vi "Demo.vi"() -> ()   [LabVIEW 2020]
uses:
  Instantiate.vi
  Flex.lvlib
panel:
  out "Timed Out?":bool
  out "Count 2":i32
  out "Count 1":i32
  out "Slow i":i32
  out "Fast i":i32
  out "Lossy Fast Timeout":bool
  out "Timeout":bool
  in  "Publish Timeout":i32
  in  "Stop 4":bool
  in  "Stop 3":bool
  in  "Stop 2":bool
  in  "Stop 1":bool
  in  "Stop":bool
  out "Lossless Timeout":dbl(graph)
  out "Lossless":dbl(graph)
  out "Lossy Slow/Wait":dbl(graph)
  out "Lossy Fast":dbl(graph)
  in  "Publish Period mS":u32=10
  in  "Slide":dbl(slide)=5.0 scale=0.0..10.0
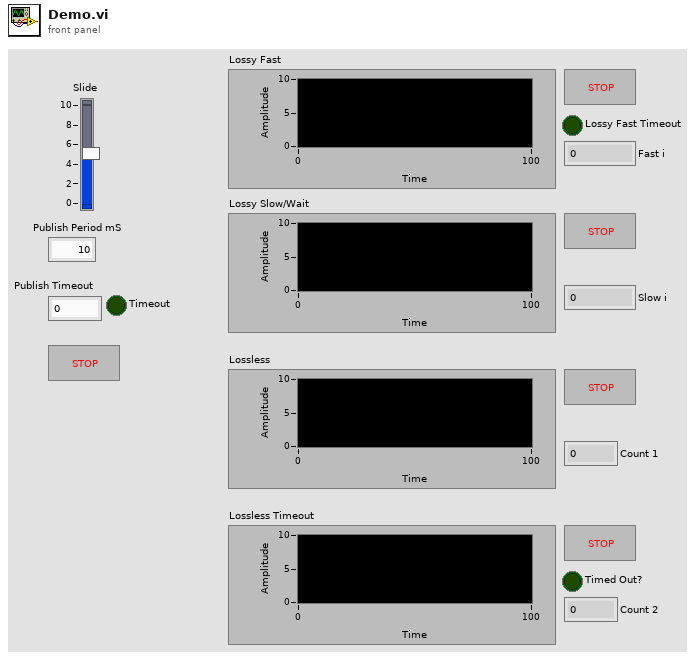
[diagram p1: front panel]
types:
  T1 = typedef "Flex.lvlib/))Channel.ctl" = refnum<queue>
  T2 = typedef "Flex.lvlib/Element.ctl" = dbl
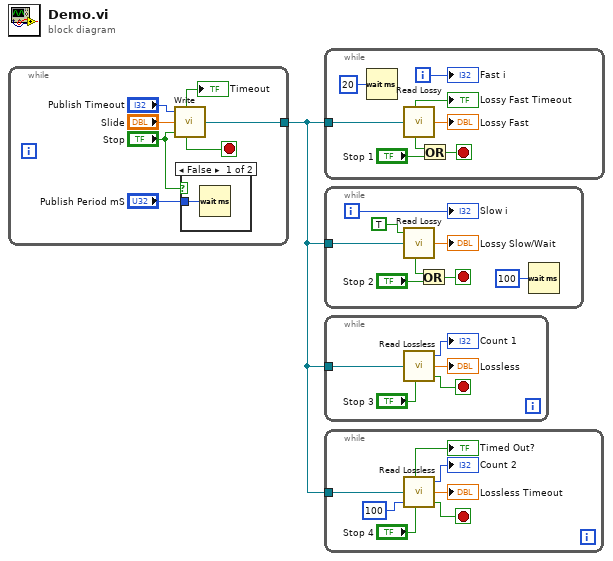
[diagram p0: block diagram]
diagram:
  n1 = while {
    tunnel: [w3] -> w1
    stop <- w4 stop-if-true
    n2 = call "Write.vi"("Timeout mS (-1)"="Publish Timeout", "element"="Slide", "Close? (F)"="Stop") -> ("Timed Out?"=→"Timeout":bool, "Closed?"=w4:bool, "channel"=w3:T1)  [unwired: 2 in]
    n3 = case shown="False" "Stop" {
      tunnel: "Publish Period mS" -> [w9 _]
      frame False {
        n4 = Wait (ms)(milliseconds to wait=w9) -> ()  [unwired: 1 out]
      }
      frame True {
      }
    }
  }
  n5 = while {
    tunnel: w1 -> [w17]
    i -> [w11]
    stop <- w12 stop-if-true
    n6 = Wait (ms)(milliseconds to wait=u32 20) -> ()  [unwired: 1 out]
    n7 = call "Read Lossy.vi"("FlexChannel"=w17) -> ("Timed Out?"=→"Lossy Fast Timeout":bool, "Closed?"=w13:bool, "Element"=→"Lossy Fast":T2)  [unwired: 4 in]
    n8 = Or(x=w13, y="Stop 1") -> (x .or. y?=w12:bool)
    "Fast i" <- w11
  }
  n9 = while {
    tunnel: w1 -> [w24]
    i -> [w19]
    stop <- w21 stop-if-true
    n10 = call "Read Lossy.vi"("Wait for Next? (F)"=TRUE, "FlexChannel"=w24) -> ("Closed?"=w22:bool, "Element"=→"Lossy Slow/Wait":T2)  [unwired: 3 in, 1 out]
    n11 = Or(x=w22, y="Stop 2") -> (x .or. y?=w21:bool)
    n12 = Wait (ms)(milliseconds to wait=u32 100) -> ()  [unwired: 1 out]
    "Slow i" <- w19
  }
  n13 = while {
    tunnel: w1 -> [w30]
    stop <- w26 stop-if-true
    n14 = call "Read Lossless.vi"("FlexChannel"=w30, "Release (F)"="Stop 3") -> ("Count"=→"Count 1":i32, "Element"=→"Lossless":T2, "Closed?"=w26:bool)  [unwired: 2 in, 1 out]
  }
  n15 = while {
    tunnel: w1 -> [w33]
    stop <- w32 stop-if-true
    n16 = call "Read Lossless.vi"("FlexChannel"=w33, "Timeout mS (-1)"=100, "Release (F)"="Stop 4") -> ("Timed Out?"=→"Timed Out?":bool, "Count"=→"Count 2":i32, "Element"=→"Lossless Timeout":T2, "Closed?"=w32:bool)  [unwired: 1 in]
  }
